vi "niRFUtil WFM Trim Waveform.vi"(8 "error in (no error)":errorcluster, 10 "Samples to Read":i32=-1, 11 "Waveform In":T1 {"y" format="%.2f"; "dx" format="%^.2e"; "x0" format="%^.2e"}) -> (0 "error out":errorcluster, 3 "Waveform Out":T1 {"y" format="%.2f"; "dx" format="%^.2e"; "x0" format="%^.2e"})   [LabVIEW 2015, in "niRFUtil.lvlib"]
uses:
  niRFUtil.lvlib
  Includes/niRFUtil INC Complex Waveform.ctl
  Includes/niRFUtil INC Complex Array.ctl
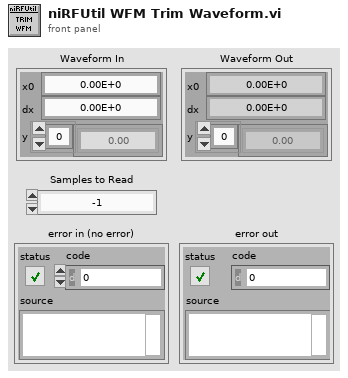
[diagram p1: front panel]
types:
  T1 = typedef "niRFUtil.lvlib/niRFUtil INC Complex Waveform.ctl" = cluster{"x0":dbl, "dx":dbl, "y":T2}
  T2 = typedef "niRFUtil.lvlib/niRFUtil INC Complex Array.ctl" = csg[]
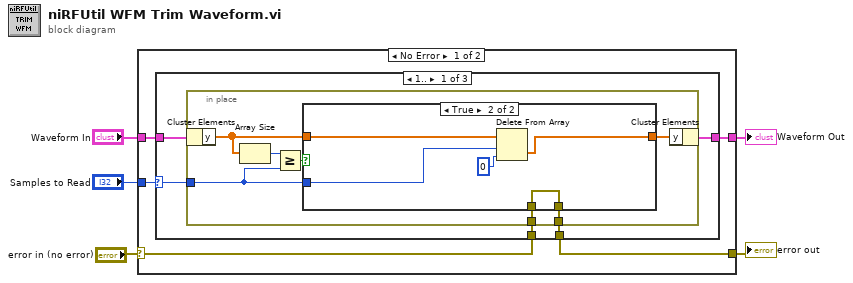
[diagram p0: block diagram]
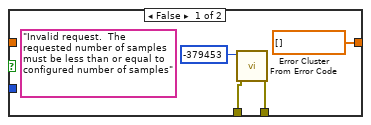
[diagram p2: hidden frame]
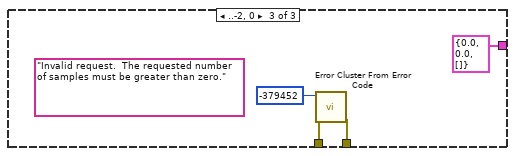
[diagram p4: hidden frame]
diagram:
  n1 = case shown="No Error" "error in (no error)" {
    selector: "error in (no error)" -> [w7 w39]
    tunnel: [w10 w38] -> w5
    tunnel: "Waveform In" -> [w9 w38]
    tunnel: "Samples to Read" -> [w8 _]
    tunnel: [w6 w39] -> w1
    frame No Error {
      n2 = case shown="1.." w8 {
        selector: w8 -> [w13 _ _]
        tunnel: w9 -> [w15 w33 _]
        tunnel: [w14 w33 T1 {"x0"=0.0, "dx"=0.0, "y"=[]} ("Waveform In")] -> w10
        tunnel: w7 -> [w12 w32 w36]
        tunnel: [w11 w32 w35] -> w6
        frame 1.. {
          n3 = in-place {
            in-place-border: w13 -> [w18]
            in-place-border: w12 -> [w17]
            in-place-border: [w16] -> w11
            n4 = in-place-cluster #1(w15) -> ("y"=w21:T2)
            n5 = Array Size(array=w21) -> (size(s)=w20:i32)
            n6 = Greater Or Equal?(x=w20, y=w18) -> (x >= y?=w19:bool)
            n7 = case shown="True" w19 {
              tunnel: [T2 [] ("y") w31] -> w22
              tunnel: w21 -> [_ w29]
              tunnel: w18 -> [_ w28]
              tunnel: w17 -> [w25 w27]
              tunnel: [w24 w27] -> w16
              frame False {
                (unwired) "Invalid request.  The requested number of samples must be less than or equal to configured number of samples"
                n8 = call <vilib>:"Error Cluster From Error Code.vi"("error in (no error)"=w25, "error code (0)"=-379453) -> ("error out"=w24:errorcluster)  [unwired: 7 in]
              }
              frame True {
                n9 = Delete From Array(array=w29, length=w28, index=0) -> (deleted portion=w31:T2)  [unwired: 1 out]
              }
            }
            n10 = in-place-cluster #1("y"=w22) -> (w14:T1)
          }
        }
        frame -1 {
        }
        frame ..-2, 0 {
          (unwired) "Invalid request.  The requested number of samples must be greater than zero."
          n11 = call <vilib>:"Error Cluster From Error Code.vi"("error in (no error)"=w36, "error code (0)"=-379452) -> ("error out"=w35:errorcluster)  [unwired: 7 in]
        }
      }
    }
    frame Error {
    }
  }
  "Waveform Out" <- w5
  "error out" <- w1
